vi "rsscope_core_global.vi"() -> ()   [LabVIEW 2014] (continued)
"Range Table"="rsscope_rngNqEq", "Read Callback"="", "Write Callback"="", "Supported Models"="", "Instrument Options"="", "Flags"=0, "Help"="Selects the operator for the MISO and MOSI pattern.\n\nAvailable Repeated Capabilities:\nTrigger: TrigA, TrigB, TrigR\r\n\nRemote-control command(s):\nTRIGger<m>:SPI:FCONdition"}, {"Level"=3, "Class Only"=FALSE, "Identifier"="RSSCOPE_ATTR_PROTOCOL_SPI_TRIGGER_MOSI_PATTERN", "Descriptive Name"="Protocol SPI Trigger MOSI Pattern", "Data Type"=2, "Command"="TRIG{Trigger}:SPI:MOS", "Access"=2, "Range Table"="", "Read Callback"="", "Write Callback"="", "Supported Models"="", "Instrument Options"="", "Flags"=0, "Help"="Specifies the pattern to be triggered on the MOSI line.\n\nAvailable Repeated Capabilities:\nTrigger: TrigA, TrigB, TrigR\r\n\nRemote-control command(s):\nTRIGger<m>:SPI:MOSipattern"}, {"Level"=3, "Class Only"=FALSE, "Identifier"="RSSCOPE_ATTR_PROTOCOL_SPI_TRIGGER_MISO_PATTERN", "Descriptive Name"="Protocol SPI Trigger MISO Pattern", "Data Type"=2, "Command"="TRIG{Trigger}:SPI:MIS", "Access"=2, "Range Table"="", "Read Callback"="", "Write Callback"="", "Supported Models"="", "Instrument Options"="", "Flags"=0, "Help"="Specifies the pattern to be triggered on the MOSI line.\n\nAvailable Repeated Capabilities:\nTrigger: TrigA, TrigB, TrigR\r\n\nRemote-control command(s):\nTRIGger<m>:SPI:MISopattern"}, {"Level"=2, "Class Only"=TRUE, "Identifier"="", "Descriptive Name"="UART", "Data Type"=0, "Command"="", "Access"=0, "Range Table"="", "Read Callback"="", "Write Callback"="", "Supported Models"="", "Instrument Options"="", "Flags"=0, "Help"="Configures UART trigger settings."}, {"Level"=3, "Class Only"=FALSE, "Identifier"="RSSCOPE_ATTR_PROTOCOL_UART_TRIGGER_MODE", "Descriptive Name"="Protocol UART Trigger Mode", "Data Type"=0, "Command"="TRIG{Trigger}:UART:TYPE", "Access"=2, "Range Table"="rsscope_rngProtocolUARTTriggerType", "Read Callback"="", "Write Callback"="", "Supported Models"="", "Instrument Options"="", "Flags"=0, "Help"="Selects the trigger type for UART analysis.\n\nAvailable Repeated Capabilities:\nTrigger: TrigA, TrigB, TrigR\r\n\nRemote-control command(s):\nTRIGger<m>:UART:TYPE"}, {"Level"=3, "Class Only"=FALSE, "Identifier"="RSSCOPE_ATTR_PROTOCOL_UART_TRIGGER_SOURCE", "Descriptive Name"="Protocol UART Trigger Source", "Data Type"=0, "Command"="TRIG{Trigger}:UART:SOUR", "Access"=2, "Range Table"="rsscope_rngProtocolUARTLine", "Read Callback"="", "Write Callback"="", "Supported Models"="", "Instrument Options"="", "Flags"=0, "Help"="Selects the transmitter or receiver line as trigger source.\n\nAvailable Repeated Capabilities:\nTrigger: TrigA, TrigB, TrigR\r\n\nRemote-control command(s):\nTRIGger<m>:UART:SOURce"}, {"Level"=3, "Class Only"=FALSE, "Identifier"="RSSCOPE_ATTR_PROTOCOL_UART_TRIGGER_DATA_PATTERN", "Descriptive Name"="Protocol UART Trigger Data Pattern", "Data Type"=2, "Command"="TRIG{Trigger}:UART:DATA", "Access"=2, "Range Table"="", "Read Callback"="", "Write Callback"="", "Supported Models"="", "Instrument Options"="", "Flags"=0, "Help"="Specifies the data pattern to be found on the specified trigger source, in bin format. Enter the words in msb first bit order.\n\nAvailable Repeated Capabilities:\nTrigger: TrigA, TrigB, TrigR\r\n\nRemote-control command(s):\nTRIGger<m>:UART:DATA"}, {"Level"=3, "Class Only"=FALSE, "Identifier"="RSSCOPE_ATTR_PROTOCOL_UART_TRIGGER_DATA_PATTERN_CONDITION", "Descriptive Name"="Protocol UART Trigger Data Pattern Condition", "Data Type"=0, "Command"="TRIG{Trigger}:UART:FCON", "Access"=2, "Range Table"="rsscope_rngProtocolUARTDataOperator", "Read Callback"="", "Write Callback"="", "Supported Models"="", "Instrument Options"="", "Flags"=0, "Help"="Selects the operator for the data pattern.\n\nAvailable Repeated Capabilities:\nTrigger: TrigA, TrigB, TrigR\r\n\nRemote-control command(s):\nTRIGger<m>:UART:FCONdition"}, {"Level"=3, "Class Only"=FALSE, "Identifier"="RSSCOPE_ATTR_PROTOCOL_UART_TRIGGER_DATA_POSITION", "Descriptive Name"="Protocol UART Trigger Data Position", "Data Type"=0, "Command"="TRIG{Trigger}:UART:DPOP", "Access"=2, "Range Table"="rsscope_rngProtocolUARTDataPosition", "Read Callback"="", "Write Callback"="", "Supported Models"="", "Instrument Options"="", "Flags"=0, "Help"="Sets the operator for the data position. You can defined an exact position, or a position range.\n\nAvailable Repeated Capabilities:\nTrigger: TrigA, TrigB, TrigR\r\n\nRemote-control command(s):\nTRIGger<m>:UART:DPOPerator"}, {"Level"=3, "Class Only"=FALSE, "Identifier"="RSSCOPE_ATTR_PROTOCOL_UART_TRIGGER_DATA_POSITION_INDEX_MIN", "Descriptive Name"="Protocol UART Trigger Data Position Index Min", "Data Type"=0, "Command"="TRIG{Trigger}:UART:DPOS", "Access"=2, "Range Table"="rsscope_rngProtocolUARTDataIndexMin", "Read Callback"="", "Write Callback"="", "Supported Models"="", "Instrument Options"="", "Flags"=0, "Help"="Sets the number of words before the first word of interest. These offset words are ignored.\n\nAvailable Repeated Capabilities:\nTrigger: TrigA, TrigB, TrigR\r\n\nRemote-control command(s):\nTRIGger<m>:UART:DPOSition"}, {"Level"=3, "Class Only"=FALSE, "Identifier"="RSSCOPE_ATTR_PROTOCOL_UART_TRIGGER_DATA_POSITION_INDEX_MAX", "Descriptive Name"="Protocol UART Trigger Data Position Index Max", "Data Type"=0, "Command"="TRIG:UART:DPTO", "Access"=2, "Range Table"="rsscope_rngProtocolUARTDataIndexMax", "Read Callback"="", "Write Callback"="", "Supported Models"="", "Instrument Options"="", "Flags"=0, "Help"="Defines the last word of interest, if  RSSCOPE_ATTR_PROTOCOL_UART_TRIGGER_DATA_POSITION \ndefines a position range.\n\nAvailable Repeated Capabilities:\nNone\n\nRemote-control command(s):\nTRIGger<m>:UART:DPTO"}, {"Level"=2, "Class Only"=TRUE, "Identifier"="", "Descriptive Name"="LIN", "Data Type"=0, "Command"="", "Access"=0, "Range Table"="", "Read Callback"="", "Write Callback"="", "Supported Models"="", "Instrument Options"="", "Flags"=0, "Help"="Configures LIN trigger settings."}, {"Level"=3, "Class Only"=FALSE, "Identifier"="RSSCOPE_ATTR_PROTOCOL_LIN_TRIGGER_MODE", "Descriptive Name"="Protocol LIN Trigger Mode", "Data Type"=0, "Command"="TRIG{Trigger}:LIN:TYPE", "Access"=2, "Range Table"="rsscope_rngProtocolLINTrigger", "Read Callback"="", "Write Callback"="", "Supported Models"="", "Instrument Options"="K0|K3", "Flags"=0, "Help"="Selects the trigger type for LIN analysis.\n\nAvailable Repeated Capabilities:\nTrigger: TrigA, TrigB, TrigR\r\n\nRemote-control command(s):\nTRIGger<m>:LIN:TYPE"}, {"Level"=3, "Class Only"=FALSE, "Identifier"="RSSCOPE_ATTR_PROTOCOL_LIN_TRIGGER_DATA_CONDITION", "Descriptive Name"="Protocol LIN Trigger Data Condition", "Data Type"=0, "Command"="TRIG{Trigger}:LIN:DLEC", "Access"=2, "Range Table"="rsscope_rngProtocolLINTriggerDataCondition", "Read Callback"="", "Write Callback"="", "Supported Models"="", "Instrument Options"="", "Flags"=0, "Help"="Sets the operator to set the data length code for triggering on LIN data. For big endian transfer direction, you can trigger on a number of bytes less than the data length of the frame, that means, on the beginning of the data pattern. For little endian transfer direction, the exact number of data bytes in the frame must be set.\n\nAvailable Repeated Capabilities:\nTrigger: TrigA, TrigB, TrigR\r\n\nRemote-control command(s):\nTRIGger<m>:LIN:DLECondition"}, {"Level"=3, "Class Only"=FALSE, "Identifier"="RSSCOPE_ATTR_PROTOCOL_LIN_TRIGGER_DATA_LENGTH", "Descriptive Name"="Protocol LIN Trigger Data Length", "Data Type"=0, "Command"="TRIG{Trigger}:LIN:DLEN", "Access"=2, "Range Table"="rsscope_rngLINDataLength", "Read Callback"="", "Write Callback"="", "Supported Models"="", "Instrument Options"="", "Flags"=0, "Help"="Sets the length of the bit pattern to be found, in bytes. For &apos;Big Endian&apos; transfer direction, you can trigger on a number of bytes less than the data length of the frame, that means, on the beginning of the data pattern. For &apos;Little Endian&apos; transfer direction, the exact number of data bytes in the frame must be set.\n\nAvailable Repeated Capabilities:\nTrigger: TrigA, TrigB, TrigR\r\n\nRemote-control command(s):\nTRIGger<m>:LIN:DLENgth"}, {"Level"=3, "Class Only"=FALSE, "Identifier"="RSSCOPE_ATTR_PROTOCOL_LIN_TRIGGER_DATA_TRANSFER", "Descriptive Name"="Protocol LIN Trigger Data Transfer", "Data Type"=0, "Command"="TRIG{Trigger}:LIN:BORD", "Access"=2, "Range Table"="rsscope_rngLINDataTransfer", "Read Callback"="", "Write Callback"="", "Supported Models"="", "Instrument Options"="", "Flags"=0, "Help"="Sets the byte order (endianess) of the data transfer. According to the standard, LIN data is transmitted in little endian transfer order.\n\nAvailable Repeated Capabilities:\nTrigger: TrigA, TrigB, TrigR\r\n\nRemote-control command(s):\nTRIGger<m>:LIN:BORDer"}, {"Level"=3, "Class Only"=TRUE, "Identifier"="", "Descriptive Name"="Data", "Data Type"=0, "Command"="", "Access"=0, "Range Table"="", "Read Callback"="", "Write Callback"="", "Supported Models"="", "Instrument Options"="", "Flags"=0, "Help"="Configures data setup."}, {"Level"=4, "Class Only"=FALSE, "Identifier"="RSSCOPE_ATTR_PROTOCOL_LIN_TRIGGER_CONDITION_DATA", "Descriptive Name"="Protocol LIN Trigger Condition Data", "Data Type"=0, "Command"="TRIG{Trigger}:LIN:DCON", "Access"=2, "Range Table"="rsscope_rngProtocolTriggerCondition", "Read Callback"="", "Write Callback"="", "Supported Models"="", "Instrument Options"="", "Flags"=0, "Help"="Sets the operator to set a specific data or an data range.\n\nAvailable Repeated Capabilities:\nTrigger: TrigA, TrigB, TrigR\r\n\nRemote-control command(s):\nTRIGger<m>:LIN:DCONdition"}, {"Level"=4, "Class Only"=FALSE, "Identifier"="RSSCOPE_ATTR_PROTOCOL_LIN_TRIGGER_PATTERN_DATA_MIN", "Descriptive Name"="Protocol LIN Trigger Pattern Data Min", "Data Type"=2, "Command"="TRIG{Trigger}:LIN:DMIN", "Access"=2, "Range Table"="", "Read Callback"="", "Write Callback"="", "Supported Models"="", "Instrument Options"="", "Flags"=0, "Help"="Sets the trigger pattern, or sets the start value of an pattern range.\n\nNote(s):\n\n(1) Valid values 1; 0; or X (any bit), use of X is restricted to the conditions &apos;Equal&apos; and &apos;Not equal&apos;.\n\n(2) Data binary pattern string consist 8 Bytes.\n\nAvailable Repeated Capabilities:\nTrigger: TrigA, TrigB, TrigR\r\n\nRemote-control command(s):\nTRIGger<m>:LIN:DMIN"}, {"Level"=4, "Class Only"=FALSE, "Identifier"="RSSCOPE_ATTR_PROTOCOL_LIN_TRIGGER_PATTERN_DATA_MAX", "Descriptive Name"="Protocol LIN Trigger Pattern Data Max", "Data Type"=2, "Command"="TRIG{Trigger}:LIN:DMAX", "Access"=2, "Range Table"="", "Read Callback"="", "Write Callback"="", "Supported Models"="", "Instrument Options"="", "Flags"=0, "Help"="Sets the end value of trigger pattern range if condition is &apos;In range&apos; and &apos;Out of range&apos; (see RSSCOPE_ATTR_PROTOCOL_LIN_TRIGGER_CONDITION).\n \nNote(s):\n(1) Valid values 1; 0; or X (any bit), use of X is restricted to the conditions &apos;Equal&apos; and &apos;Not equal&apos;.\n\n(2) Data binary pattern string consist 8 Bytes.\n\nAvailable Repeated Capabilities:\nTrigger: TrigA, TrigB, TrigR\r\n\nRemote-control command(s):\nTRIGger<m>:LIN:DMAX"}, {"Level"=3, "Class Only"=TRUE, "Identifier"="", "Descriptive Name"="Identifier", "Data Type"=0, "Command"="", "Access"=0, "Range Table"="", "Read Callback"="", "Write Callback"="", "Supported Models"="", "Instrument Options"="", "Flags"=0, "Help"="Configures identifier setup."}, {"Level"=4, "Class Only"=FALSE, "Identifier"="RSSCOPE_ATTR_PROTOCOL_LIN_TRIGGER_IDENTIFIER_CONDITION", "Descriptive Name"="Protocol LIN Trigger Identifier Condition", "Data Type"=0, "Command"="TRIG{Trigger}:LIN:ICON", "Access"=2, "Range Table"="rsscope_rngProtocolTriggerCondition", "Read Callback"="", "Write Callback"="", "Supported Models"="", "Instrument Options"="", "Flags"=0, "Help"="Sets the operator to set a specific identifier or an identifier range.\n\nAvailable Repeated Capabilities:\nTrigger: TrigA, TrigB, TrigR\r\n\nRemote-control command(s):\nTRIGger<m>:LIN:ICONdition"}, {"Level"=4, "Class Only"=FALSE, "Identifier"="RSSCOPE_ATTR_PROTOCOL_LIN_TRIGGER_PATTERN_IDENTIFIER_MIN", "Descriptive Name"="Protocol LIN Trigger Pattern Identifier Min", "Data Type"=2, "Command"="TRIG{Trigger}:LIN:IMIN", "Access"=2, "Range Table"="", "Read Callback"="", "Write Callback"="", "Supported Models"="", "Instrument Options"="", "Flags"=0, "Help"="Sets the trigger pattern, or sets the start value of an pattern range.\n\nNote(s):\n\n(1) Valid values 1; 0; or X (any bit), use of X is restricted to the conditions &apos;Equal&apos; and &apos;Not equal&apos;.\n\n(2) ID binary pattern string consist 6 bits.\n\nAvailable Repeated Capabilities:\nTrigger: TrigA, TrigB, TrigR\r\n\nRemote-control command(s):\nTRIGger<m>:LIN:IMIN"}, {"Level"=4, "Class Only"=FALSE, "Identifier"="RSSCOPE_ATTR_PROTOCOL_LIN_TRIGGER_PATTERN_IDENTIFIER_MAX", "Descriptive Name"="Protocol LIN Trigger Pattern Identifier Max", "Data Type"=2, "Command"="TRIG{Trigger}:LIN:IMAX", "Access"=2, "Range Table"="", "Read Callback"="", "Write Callback"="", "Supported Models"="", "Instrument Options"="", "Flags"=0, "Help"="Sets the end value of trigger pattern range if condition is &apos;In range&apos; and &apos;Out of range&apos; (see RSSCOPE_ATTR_PROTOCOL_LIN_TRIGGER_CONDITION).\n \nNote(s):\n(1) Valid values 1; 0; or X (any bit), use of X is restricted to the conditions &apos;Equal&apos; and &apos;Not equal&apos;.\n\n(2) ID binary pattern string consist 6 bits.\n\nAvailable Repeated Capabilities:\nTrigger: TrigA, TrigB, TrigR\r\n\nRemote-control command(s):\nTRIGger<m>:LIN:IMAX"}, {"Level"=3, "Class Only"=TRUE, "Identifier"="", "Descriptive Name"="OR Slot", "Data Type"=0, "Command"="", "Access"=0, "Range Table"="", "Read Callback"="", "Write Callback"="", "Supported Models"="", "Instrument Options"="", "Flags"=0, "Help"="Sets the trigger to a combination of up to four identifiers. Enter the patterns in the &apos;Frame\nID&apos; fields. In binary and hex format, characters 1, 0, and X (don&apos;t care) are allowed. For\neach identifier pattern to be triggered on, enable &apos;Monitor&apos;."}, {"Level"=4, "Class Only"=FALSE, "Identifier"="RSSCOPE_ATTR_PROTOCOL_LIN_TRIGGER_ADDRESS_OR_STATE", "Descriptive Name"="Protocol LIN Trigger Address OR State", "Data Type"=3, "Command"="TRIG{Trigger}:LIN:IDOR{ORSlot}:ENAB", "Access"=2, "Range Table"="", "Read Callback"="", "Write Callback"="", "Supported Models"="", "Instrument Options"="K0|K3", "Flags"=2, "Help"="If set to &apos;On&apos; the indicated ADOR address is included in the &apos;identifier OR&apos; trigger condition.\n\nAvailable Repeated Capabilities:\nTrigger: TrigA, TrigB, TrigR\r\nORSlot: ORSlot1, ORSlot2, ORSlot3, ORSlot4\r\n\nRemote-control command(s):\nTRIGger<m>:LIN:IDOR<n>:ENABle"}, {"Level"=4, "Class Only"=FALSE, "Identifier"="RSSCOPE_ATTR_PROTOCOL_LIN_TRIGGER_ADDRESS_OR", "Descriptive Name"="Protocol LIN Trigger Address OR", "Data Type"=2, "Command"="TRIG{Trigger}:LIN:IDOR{ORSlot}", "Access"=2, "Range Table"="", "Read Callback"="", "Write Callback"="", "Supported Models"="", "Instrument Options"="K0|K3", "Flags"=0, "Help"="Sets the pattern of the indicated IDOR identifier in the &apos;identifier OR&apos; trigger condition.\n\nValid Values: \nBinary pattern string consisting bits of 1; 0; or X (any bit).\n\nAvailable Repeated Capabilities:\nTrigger: TrigA, TrigB, TrigR\r\nORSlot: ORSlot1, ORSlot2, ORSlot3, ORSlot4\r\n\nRemote-control command(s):\nTRIGger<m>:LIN:IDOR<n>[:VALue]"}, {"Level"=3, "Class Only"=TRUE, "Identifier"="", "Descriptive Name"="Error Conditions", "Data Type"=0, "Command"="", "Access"=0, "Range Table"="", "Read Callback"="", "Write Callback"="", "Supported Models"="", "Instrument Options"="", "Flags"=0, "Help"="Triggers if one or more of the following errors occur: Checksum error, Identifier parity error, Sync error."}, {"Level"=4, "Class Only"=FALSE, "Identifier"="RSSCOPE_ATTR_PROTOCOL_LIN_TRIGGER_CHECKSUM_ERROR", "Descriptive Name"="Protocol LIN Trigger Checksum Error", "Data Type"=3, "Command"="TRIG{Trigger}:LIN:CHKS", "Access"=2, "Range Table"="", "Read Callback"="", "Write Callback"="", "Supported Models"="", "Instrument Options"="", "Flags"=0, "Help"="This attribute configures conditions for Error Condition trigger. It&apos;s possible trigger on CRC Error.\n\nAvailable Repeated Capabilities:\nTrigger: TrigA, TrigB, TrigR\r\n\nRemote-control command(s):\nTRIGger<m>:LIN:CHKSerror"}, {"Level"=4, "Class Only"=FALSE, "Identifier"="RSSCOPE_ATTR_PROTOCOL_LIN_TRIGGER_CRC_ERROR_PATTERN", "Descriptive Name"="Protocol LIN Trigger CRC Error Pattern", "Data Type"=2, "Command"="TRIG{Trigger}:LIN:ERRP", "Access"=2, "Range Table"="", "Read Callback"="", "Write Callback"="", "Supported Models"="", "Instrument Options"="K0|K3", "Flags"=0, "Help"="Sets bit pattern of the slave identifier (&apos;ID&apos;).\n\nValid Values: \nBinary pattern string consisting 1; 0; or X (any bit).\n\nAvailable Repeated Capabilities:\nTrigger: TrigA, TrigB, TrigR\r\n\nRemote-control command(s):\nTRIGger<m>:LIN:ERRPattern"}, {"Level"=4, "Class Only"=FALSE, "Identifier"="RSSCOPE_ATTR_PROTOCOL_LIN_TRIGGER_CRC_ERROR_DATA_LENGTH", "Descriptive Name"="Protocol LIN Trigger CRC Error Data Length", "Data Type"=0, "Command"="TRIG{Trigger}:LIN:CRCD", "Access"=2, "Range Table"="rsscope_rngLINTriggerCRCErrDataLength", "Read Callback"="", "Write Callback"="", "Supported Models"="", "Instrument Options"="K0|K3", "Flags"=0, "Help"="Sets the number of data bytes to trigger on CRC errors.\n\nAvailable Repeated Capabilities:\nTrigger: TrigA, TrigB, TrigR\r\n\nRemote-control command(s):\nTRIGger<m>:LIN:CRCDatalen"}, {"Level"=4, "Class Only"=FALSE, "Identifier"="RSSCOPE_ATTR_PROTOCOL_LIN_TRIGGER_CRC_STANDARD", "Descriptive Name"="Protocol LIN Trigger CRC Standard", "Data Type"=0, "Command"="TRIG{Trigger}:LIN:STAN", "Access"=2, "Range Table"="rsscope_rngProtocolLINTriggerCRCStandard", "Read Callback"="", "Write Callback"="", "Supported Models"="", "Instrument Options"="", "Flags"=0, "Help"="Sets the LIN standard to trigger on CRC errors.\n\nAvailable Repeated Capabilities:\nTrigger: TrigA, TrigB, TrigR\r\n\nRemote-control command(s):\nTRIGger<m>:LIN:STANdard"}, {"Level"=4, "Class Only"=FALSE, "Identifier"="RSSCOPE_ATTR_PROTOCOL_LIN_TRIGGER_IDENTIFIER_PARITY_ERROR", "Descriptive Name"="Protocol LIN Trigger Identifier Parity Error", "Data Type"=3, "Command"="TRIG{Trigger}:LIN:IPER", "Access"=2, "Range Table"="", "Read Callback"="", "Write Callback"="", "Supported Models"="", "Instrument Options"="", "Flags"=0, "Help"="Triggers if an error occurs in the identifier parity bits. These are the bits 6 and 7 of the\nidentifier.\n\nAvailable Repeated Capabilities:\nTrigger: TrigA, TrigB, TrigR\r\n\nRemote-control command(s):\nTRIGger<m>:LIN:IPERror"}, {"Level"=4, "Class Only"=FALSE, "Identifier"="RSSCOPE_ATTR_PROTOCOL_LIN_TRIGGER_SYNC_ERROR", "Descriptive Name"="Protocol LIN Trigger Sync Error", "Data Type"=3, "Command"="TRIG{Trigger}:LIN:SYER", "Access"=2, "Range Table"="", "Read Callback"="", "Write Callback"="", "Supported Models"="", "Instrument Options"="", "Flags"=0, "Help"="Triggers if a synchronization error occurs.\n\nAvailable Repeated Capabilities:\nTrigger: TrigA, TrigB, TrigR\r\n\nRemote-control command(s):\nTRIGger<m>:LIN:SYERror"}, {"Level"=2, "Class Only"=TRUE, "Identifier"="", "Descriptive Name"="CAN", "Data Type"=0, "Command"="", "Access"=0, "Range Table"="", "Read Callback"="", "Write Callback"="", "Supported Models"="", "Instrument Options"="", "Flags"=0, "Help"="Configures CAN trigger settings."}, {"Level"=3, "Class Only"=FALSE, "Identifier"="RSSCOPE_ATTR_PROTOCOL_CAN_TRIGGER_MODE", "Descriptive Name"="Protocol CAN Trigger Mode", "Data Type"=0, "Command"="TRIG{Trigger}:CAN:TYPE", "Access"=2, "Range Table"="rsscope_rngProtocolCANTriggMode", "Read Callback"="", "Write Callback"="", "Supported Models"="", "Instrument Options"="K0|K3", "Flags"=0, "Help"="Selects the trigger type for CAN analysis.\n\nAvailable Repeated Capabilities:\nTrigger: TrigA, TrigB, TrigR\r\n\nRemote-control command(s):\nTRIGger<m>:CAN:TYPE"}, {"Level"=3, "Class Only"=FALSE, "Identifier"="RSSCOPE_ATTR_PROTOCOL_CAN_TRIGGER_FRAME_TYPE", "Descriptive Name"="Protocol CAN Trigger Frame Type", "Data Type"=0, "Command"="TRIG{Trigger}:CAN:FTYP", "Access"=2, "Range Table"="rsscope_rngProtocolCANTriggFrameType", "Read Callback"="", "Write Callback"="", "Supported Models"="", "Instrument Options"="K0|K3", "Flags"=0, "Help"="Selects the frame type which will be used as trigger condition when trigger mode is set to &apos;Frame Type&apos; (see RSSCOPE_ATTR_PROTOCOL_CAN_TRIGGER_MODE)\n\nAvailable Repeated Capabilities:\nTrigger: TrigA, TrigB, TrigR\r\n\nRemote-control command(s):\nTRIGger<m>:CAN:FTYPe"}, {"Level"=3, "Class Only"=FALSE, "Identifier"="RSSCOPE_ATTR_PROTOCOL_CAN_TRIGGER_STANDARD", "Descriptive Name"="Protocol CAN Trigger Standard", "Data Type"=0, "Command"="TRIG{Trigger}:CAN:FDAT:STAN", "Access"=2, "Range Table"="rsscope_rngCANStandard", "Read Callback"="", "Write Callback"="", "Supported Models"="", "Instrument Options"="K9", "Flags"=0, "Help"="Selects the CAN standard. Use ANY if the standard of the signal is unknown.\n\nAvailable Repeated Capabilities:\nTrigger: TrigA, TrigB, TrigR\r\n\nRemote-control command(s):\nTRIGger<m>:CAN:FDATa:STANdard"}, {"Level"=3, "Class Only"=FALSE, "Identifier"="RSSCOPE_ATTR_PROTOCOL_CAN_TRIGGER_ID_TYPE", "Descriptive Name"="Protocol CAN Trigger ID Type", "Data Type"=0, "Command"="TRIG{Trigger}:CAN:ITYP", "Access"=2, "Range Table"="rsscope_rngProtocolCANIDType", "Read Callback"="", "Write Callback"="", "Supported Models"="", "Instrument Options"="K0|K3", "Flags"=0, "Help"="Selects the format of data and remote frames.\n\nAvailable Repeated Capabilities:\nTrigger: TrigA, TrigB, TrigR\r\n\nRemote-control command(s):\nTRIGger<m>:CAN:ITYPe"}, {"Level"=3, "Class Only"=FALSE, "Identifier"="RSSCOPE_ATTR_PROTOCOL_CAN_TRIGGER_FD_BITS_FDF", "Descriptive Name"="Protocol CAN Trigger FD Bits FDF", "Data Type"=0, "Command"="TRIG{Trigger}:CAN:FDAT:FDF", "Access"=2, "Range Table"="rsscope_rngCANFDBits", "Read Callback"="", "Write Callback"="", "Supported Models"="", "Instrument Options"="", "Flags"=0, "Help"="Specifies the CAN FD frame format. It corresponds to the EDL bit (extended data length), which only exists in CAN FD format.\n\nAvailable Repeated Capabilities:\nTrigger: TrigA, TrigB, TrigR\r\n\nRemote-control command(s):\nTRIGger<m>:CAN:FDATa:FDF"}, {"Level"=3, "Class Only"=FALSE, "Identifier"="RSSCOPE_ATTR_PROTOCOL_CAN_TRIGGER_FD_BITS_BRS", "Descriptive Name"="Protocol CAN Trigger FD Bits BRS", "Data Type"=0, "Command"="TRIG{Trigger}:CAN:FDAT:BRS", "Access"=2, "Range Table"="rsscope_rngCANFDBitRS", "Read Callback"="", "Write Callback"="", "Supported Models"="", "Instrument Options"="", "Flags"=0, "Help"="Sets the bit rate switch bit.\n\nAvailable Repeated Capabilities:\nTrigger: TrigA, TrigB, TrigR\r\n\nRemote-control command(s):\nTRIGger<m>:CAN:FDATa:BRS"}, {"Level"=3, "Class Only"=FALSE, "Identifier"="RSSCOPE_ATTR_PROTOCOL_CAN_TRIGGER_FD_BITS_ESI", "Descriptive Name"="Protocol CAN Trigger FD Bits ESI", "Data Type"=0, "Command"="TRIG{Trigger}:CAN:FDAT:ESI", "Access"=2, "Range Table"="rsscope_rngCANFDBits", "Read Callback"="", "Write Callback"="", "Supported Models"="", "Instrument Options"="", "Flags"=0, "Help"="Sets the error state indicator bit.\n\nAvailable Repeated Capabilities:\nTrigger: TrigA, TrigB, TrigR\r\n\nRemote-control command(s):\nTRIGger<m>:CAN:FDATa:ESI"}, {"Level"=3, "Class Only"=FALSE, "Identifier"="RSSCOPE_ATTR_PROTOCOL_CAN_TRIGGER_FRAME_ENDIANNESS", "Descriptive Name"="Protocol CAN Trigger Frame Endianness", "Data Type"=0, "Command"="TRIG{Trigger}:CAN:BORD", "Access"=2, "Range Table"="rsscope_rngProtocolCANEndianness", "Read Callback"="", "Write Callback"="", "Supported Models"="", "Instrument Options"="K0|K3", "Flags"=0, "Help"="Selects the byte order (endianness) of the data transfer.\n\nAvailable Repeated Capabilities:\nTrigger: TrigA, TrigB, TrigR\r\n\nRemote-control command(s):\nTRIGger<m>:CAN:BORDer"}, {"Level"=3, "Class Only"=TRUE, "Identifier"="", "Descriptive Name"="Data", "Data Type"=0, "Command"="", "Access"=0, "Range Table"="", "Read Callback"="", "Write Callback"="", "Supported Models"="", "Instrument Options"="", "Flags"=0, "Help"="Configures Trigger CAN data."}, {"Level"=4, "Class Only"=FALSE, "Identifier"="RSSCOPE_ATTR_PROTOCOL_CAN_TRIGGER_DATA_CONDITION", "Descriptive Name"="Protocol CAN Trigger Data Condition", "Data Type"=0, "Command"="TRIG{Trigger}:CAN:DCON", "Access"=2, "Range Table"="rsscope_rngProtocolTriggerCondition", "Read Callback"="", "Write Callback"="", "Supported Models"="", "Instrument Options"="", "Flags"=0, "Help"="Sets the operator to set a specific data pattern or a data pattern range.\n\nAvailable Repeated Capabilities:\nTrigger: TrigA, TrigB, TrigR\r\n\nRemote-control command(s):\nTRIGger<m>:CAN:DCONdition"}, {"Level"=4, "Class Only"=FALSE, "Identifier"="RSSCOPE_ATTR_PROTOCOL_CAN_TRIGGER_PATTERN_DATA_MIN", "Descriptive Name"="Protocol CAN Trigger Pattern Data Min", "Data Type"=2, "Command"="TRIG{Trigger}:CAN:DMIN", "Access"=2, "Range Table"="", "Read Callback"="", "Write Callback"="", "Supported Models"="", "Instrument Options"="", "Flags"=0, "Help"="Specifies a data pattern, or sets the start value of a data pattern range.\n\nAvailable Repeated Capabilities:\nTrigger: TrigA, TrigB, TrigR\r\n\nRemote-control command(s):\nTRIGger<m>:CAN:DMIN"}, {"Level"=4, "Class Only"=FALSE, "Identifier"="RSSCOPE_ATTR_PROTOCOL_CAN_TRIGGER_PATTERN_DATA_MAX", "Descriptive Name"="Protocol CAN Trigger Pattern Data Max", "Data Type"=2, "Command"="TRIG{Trigger}:CAN:DMAX", "Access"=2, "Range Table"="", "Read Callback"="", "Write Callback"="", "Supported Models"="", "Instrument Options"="", "Flags"=0, "Help"="Sets the end value of an data range.\n\nAvailable Repeated Capabilities:\nTrigger: TrigA, TrigB, TrigR\r\n\nRemote-control command(s):\nTRIGger<m>:CAN:DMAX"}, {"Level"=4, "Class Only"=FALSE, "Identifier"="RSSCOPE_ATTR_PROTOCOL_CAN_TRIGGER_DLC_CONDITION", "Descriptive Name"="Protocol CAN Trigger DLC Condition", "Data Type"=0, "Command"="TRIG{Trigger}:CAN:DLCC", "Access"=2, "Range Table"="RsScope_rngProtocolCANTriggerDLCCondition", "Read Callback"="", "Write Callback"="", "Supported Models"="", "Instrument Options"="", "Flags"=0, "Help"="Operator to set the data length code for triggering on CAN data. For big endian transfer direction, you can trigger on a number of bytes less than the DLC of the frame, that means, on the beginning of the data pattern. For little endian transfer direction, the exact number of data bytes in the frame must be set.\n\nAvailable Repeated Capabilities:\nTrigger: TrigA, TrigB, TrigR\r\n\nRemote-control command(s):\nTRIGger<m>:CAN:DLCCondition"}, {"Level"=4, "Class Only"=FALSE, "Identifier"="RSSCOPE_ATTR_PROTOCOL_CAN_TRIGGER_DLC", "Descriptive Name"="Protocol CAN Trigger DLC", "Data Type"=0, "Command"="TRIG{Trigger}:CAN:DLC", "Access"=2, "Range Table"="RsScope_rngProtocolCANTriggerDLC", "Read Callback"="", "Write Callback"="", "Supported Models"="", "Instrument Options"="", "Flags"=0, "Help"="Sets the Data Length Code, the number of data bytes to be found.\n\nAvailable Repeated Capabilities:\nTrigger: TrigA, TrigB, TrigR\r\n\nRemote-control command(s):\nTRIGger<m>:CAN:DLC"}, {"Level"=4, "Class Only"=FALSE, "Identifier"="RSSCOPE_ATTR_PROTOCOL_CAN_TRIGGER_NUMBER_OF_DATA_BYTES", "Descriptive Name"="Protocol CAN Trigger Number Of Data Bytes", "Data Type"=0, "Command"="TRIG{Trigger}:CAN:NDBY?", "Access"=0, "Range Table"="", "Read Callback"="", "Write Callback"="", "Supported Models"="", "Instrument Options"="K3", "Flags"=0, "Help"="Returns the number of data bytes defined by DLC. DLC and NDB are different in CAN FD for DLCs > 8.\n\nAvailable Repeated Capabilities:\nTrigger: TrigA, TrigB, TrigR\r\n\nRemote-control command(s):\nTRIGger<m>:CAN:NDBYtes?"}, {"Level"=4, "Class Only"=FALSE, "Identifier"="RSSCOPE_ATTR_PROTOCOL_CAN_TRIGGER_POSITION_CONDITION", "Descriptive Name"="Protocol CAN Trigger Position Condition", "Data Type"=0, "Command"="TRIG{Trigger}:CAN:FDAT:DPOP", "Access"=2, "Range Table"="rsscope_rngProtocolCANPositionCondition", "Read Callback"="", "Write Callback"="", "Supported Models"="", "Instrument Options"="K9", "Flags"=0, "Help"="Sets the operator to define an exact position or a data range where the instrument looks for the specified data pattern.\n\nAvailable Repeated Capabilities:\nTrigger: TrigA, TrigB, TrigR\r\n\nRemote-control command(s):\nTRIGger<m>:CAN:FDATa:DPOPerator"}, {"Level"=4, "Class Only"=FALSE, "Identifier"="RSSCOPE_ATTR_PROTOCOL_CAN_TRIGGER_POSITION_MIN", "Descriptive Name"="Protocol CAN Trigger Position Min", "Data Type"=0, "Command"="TRIG{Trigger}:CAN:FDAT:DPOS", "Access"=2, "Range Table"="rsscope_rngCANPositionMin", "Read Callback"="", "Write Callback"="", "Supported Models"="", "Instrument Options"="K9", "Flags"=0, "Help"="Defines the number of the first data byte at which the data pattern may start.\n\nAvailable Repeated Capabilities:\nTrigger: TrigA, TrigB, TrigR\r\n\nRemote-control command(s):\nTRIGger<m>:CAN:FDATa:DPOSition"}, {"Level"=4, "Class Only"=FALSE, "Identifier"="RSSCOPE_ATTR_PROTOCOL_CAN_TRIGGER_POSITION_MAX", "Descriptive Name"="Protocol CAN Trigger Position Max", "Data Type"=0, "Command"="TRIG{Trigger}:CAN:FDAT:DPTO", "Access"=2, "Range Table"="rsscope_rngCANPositionMax", "Read Callback"="", "Write Callback"="", "Supported Models"="", "Instrument Options"="K9", "Flags"=0, "Help"="Sets the number of the last byte at which the required data pattern may start.\n\nAvailable Repeated Capabilities:\nTrigger: TrigA, TrigB, TrigR\r\n\nRemote-control command(s):\nTRIGger<m>:CAN:FDATa:DPTO"}, {"Level"=3, "Class Only"=TRUE, "Identifier"="", "Descriptive Name"="Identifier", "Data Type"=0, "Command"="", "Access"=0, "Range Table"="", "Read Callback"="", "Write Callback"="", "Supported Models"="", "Instrument Options"="", "Flags"=0, "Help"="Configures trigger CAN identifier."}, {"Level"=4, "Class Only"=FALSE, "Identifier"="RSSCOPE_ATTR_PROTOCOL_CAN_TRIGGER_IDENTIFIER_CONDITION", "Descriptive Name"="Protocol CAN Trigger Identifier Condition", "Data Type"=0, "Command"="TRIG{Trigger}:CAN:ICON", "Access"=2, "Range Table"="rsscope_rngProtocolTriggerCondition", "Read Callback"="", "Write Callback"="", "Supported Models"="", "Instrument Options"="", "Flags"=0, "Help"="Sets the operator to set a specific identifier or an identifier range.\n\nAvailable Repeated Capabilities:\nTrigger: TrigA, TrigB, TrigR\r\n\nRemote-control command(s):\nTRIGger<m>:CAN:ICONdition"}, {"Level"=4, "Class Only"=FALSE, "Identifier"="RSSCOPE_ATTR_PROTOCOL_CAN_TRIGGER_PATTERN_IDENTIFIER_MIN", "Descriptive Name"="Protocol CAN Trigger Pattern Identifier Min", "Data Type"=2, "Command"="TRIG{Trigger}:CAN:IMIN", "Access"=2, "Range Table"="", "Read Callback"="", "Write Callback"="", "Supported Models"="", "Instrument Options"="", "Flags"=0, "Help"="Specifies a message identifier pattern, or sets the start value of an identifier range.\n\nAvailable Repeated Capabilities:\nTrigger: TrigA, TrigB, TrigR\r\n\nRemote-control command(s):\nTRIGger<m>:CAN:IMIN"}, {"Level"=4, "Class Only"=FALSE, "Identifier"="RSSCOPE_ATTR_PROTOCOL_CAN_TRIGGER_PATTERN_IDENTIFIER_MAX", "Descriptive Name"="Protocol CAN Trigger Pattern Identifier Max", "Data Type"=2, "Command"="TRIG{Trigger}:CAN:IMAX", "Access"=2, "Range Table"="", "Read Callback"="", "Write Callback"="", "Supported Models"="", "Instrument Options"="", "Flags"=0, "Help"="Sets the end value of an identifier range.\n\nAvailable Repeated Capabilities:\nTrigger: TrigA, TrigB, TrigR\r\n\nRemote-control command(s):\nTRIGger<m>:CAN:IMAX"}, {"Level"=3, "Class Only"=TRUE, "Identifier"="", "Descriptive Name"="Error Conditions", "Data Type"=0, "Command"="", "Access"=0, "Range Table"="", "Read Callback"="", "Write Callback"="", "Supported Models"="", "Instrument Options"="", "Flags"=0, "Help"="If a CAN detects a bit stuffing error, form error, or ack error, it transmits an error flag at the next bit. The R&S RTO detects errors in the message and triggers on these errors even if no CAN node sends an error flag."}, {"Level"=4, "Class Only"=FALSE, "Identifier"="RSSCOPE_ATTR_PROTOCOL_CAN_TRIGGER_CHECKSUM_ERROR", "Descriptive Name"="Protocol CAN Trigger Checksum Error", "Data Type"=3, "Command"="TRIG{Trigger}:CAN:CRC", "Access"=2, "Range Table"="", "Read Callback"="", "Write Callback"="", "Supported Models"="", "Instrument Options"="", "Flags"=0, "Help"="Triggers on CRC errors. A CRC error occurs when the CRC calculated by the receiver differs from the received value in the CRC sequence.\n\nAvailable Repeated Capabilities:\nTrigger: TrigA, TrigB, TrigR\r\n\nRemote-control command(s):\nTRIGger<m>:CAN:CRCerror"}, {"Level"=4, "Class Only"=FALSE, "Identifier"="RSSCOPE_ATTR_PROTOCOL_CAN_TRIGGER_BIT_STUFFING_ERROR", "Descriptive Name"="Protocol CAN Trigger Bit Stuffing Error", "Data Type"=3, "Command"="TRIG{Trigger}:CAN:BITS", "Access"=2, "Range Table"="", "Read Callback"="", "Write Callback"="", "Supported Models"="", "Instrument Options"="", "Flags"=0, "Help"="Triggers if astuff error occurs - when the 6th consecutive equal bit level in the mentioned fields is detected.\n\nAvailable Repeated Capabilities:\nTrigger: TrigA, TrigB, TrigR\r\n\nRemote-control command(s):\nTRIGger<m>:CAN:BITSterror"}, {"Level"=4, "Class Only"=FALSE, "Identifier"="RSSCOPE_ATTR_PROTOCOL_CAN_TRIGGER_FORM_ERROR", "Descriptive Name"="Protocol CAN Trigger Form Error", "Data Type"=3, "Command"="TRIG{Trigger}:CAN:FORM", "Access"=2, "Range Table"="", "Read Callback"="", "Write Callback"="", "Supported Models"="", "Instrument Options"="", "Flags"=0, "Help"="Triggers when a fixed-form bit field contains one or more illegal bits.\n\nAvailable Repeated Capabilities:\nTrigger: TrigA, TrigB, TrigR\r\n\nRemote-control command(s):\nTRIGger<m>:CAN:FORMerror"}, {"Level"=4, "Class Only"=FALSE, "Identifier"="RSSCOPE_ATTR_PROTOCOL_CAN_TRIGGER_ACK_ERROR", "Descriptive Name"="Protocol CAN Trigger Ack Error", "Data Type"=3, "Command"="TRIG{Trigger}:CAN:ACK", "Access"=2, "Range Table"="", "Read Callback"="", "Write Callback"="", "Supported Models"="", "Instrument Options"="", "Flags"=0, "Help"="Triggers when the transmitter does not receive an acknowledgment - a dominant bit during the Ack Slot.\n\nAvailable Repeated Capabilities:\nTrigger: TrigA, TrigB, TrigR\r\n\nRemote-control command(s):\nTRIGger<m>:CAN:ACKerror"}, {"Level"=4, "Class Only"=FALSE, "Identifier"="RSSCOPE_ATTR_PROTOCOL_CAN_TRIGGER_STUFF_COUNT_ERROR", "Descriptive Name"="Protocol CAN Trigger Stuff Count Error", "Data Type"=3, "Command"="TRIG{Trigger}:CAN:FDAT:SCER", "Access"=2, "Range Table"="", "Read Callback"="", "Write Callback"="", "Supported Models"="", "Instrument Options"="K3", "Flags"=0, "Help"="Triggers on stuff count errors. A stuff count error occurs if th received stuff count value does not match the value calculated from the own stuff bit count.\n\nAvailable Repeated Capabilities:\nTrigger: TrigA, TrigB, TrigR\r\n\nRemote-control command(s):\nTRIGger<m>:CAN:FDATa:SCERror"}, {"Level"=3, "Class Only"=TRUE, "Identifier"="", "Descriptive Name"="Symbolic", "Data Type"=0, "Command"="", "Access"=0, "Range Table"="", "Read Callback"="", "Write Callback"="", "Supported Models"="", "Instrument Options"="", "Flags"=0, "Help"="This class configures symbolic trigger."}, {"Level"=4, "Class Only"=FALSE, "Identifier"="RSSCOPE_ATTR_PROTOCOL_CAN_SYMBOLIC_TRIGGER_MESSAGE", "Descriptive Name"="Protocol CAN Symbolic Trigger Message", "Data Type"=2, "Command"="TRIG{Trigger}:CAN:SYMB:MSGV", "Access"=2, "Range Table"="", "Read Callback"="", "Write Callback"="", "Supported Models"="", "Instrument Options"="", "Flags"=0, "Help"="Sets the message to be triggered or searched for.\n\nAvailable Repeated Capabilities:\nTrigger: TrigA, TrigB, TrigR\r\n\nRemote-control command(s):\nTRIGger<m>:CAN:SYMBolic:MSGValue"}, {"Level"=4, "Class Only"=FALSE, "Identifier"="RSSCOPE_ATTR_PROTOCOL_CAN_SYMBOLIC_TRIGGER_ON_SIGNAL", "Descriptive Name"="Protocol CAN Symbolic Trigger On Signal", "Data Type"=3, "Command"="TRIG{Trigger}:CAN:SYMB:TSIG", "Access"=2, "Range Table"="", "Read Callback"="", "Write Callback"="", "Supported Models"="", "Instrument Options"="", "Flags"=0, "Help"="Enables the trigger on a specific signal value that is part of the selected message.\n\nAvailable Repeated Capabilities:\nTrigger: TrigA, TrigB, TrigR\r\n\nRemote-control command(s):\nTRIGger<m>:CAN:SYMBolic:TSIGnals"}, {"Level"=4, "Class Only"=FALSE, "Identifier"="RSSCOPE_ATTR_PROTOCOL_CAN_SYMBOLIC_TRIGGER_SIGNAL_VALUE", "Descriptive Name"="Protocol CAN Symbolic Trigger Signal Value", "Data Type"=2, "Command"="TRIG{Trigger}:CAN:SYMB:SIGV", "Access"=2, "Range Table"="", "Read Callback"="", "Write Callback"="", "Supported Models"="", "Instrument Options"="", "Flags"=0, "Help"="Sets the signal name to be triggered or searched for.\n\nAvailable Repeated Capabilities:\nTrigger: TrigA, TrigB, TrigR\r\n\nRemote-control command(s):\nTRIGger<m>:CAN:SYMBolic:SIGValue"}, {"Level"=4, "Class Only"=FALSE, "Identifier"="RSSCOPE_ATTR_PROTOCOL_CAN_SYMBOLIC_TRIGGER_SIGNAL_MIN", "Descriptive Name"="Protocol CAN Symbolic Trigger Signal Min", "Data Type"=1, "Command"="TRIG{Trigger}:CAN:SYMB:DMIN", "Access"=2, "Range Table"="", "Read Callback"="", "Write Callback"="", "Supported Models"="", "Instrument Options"="", "Flags"=0, "Help"="Defines the minimum data value of the signal.\n\nAvailable Repeated Capabilities:\nTrigger: TrigA, TrigB, TrigR\r\n\nRemote-control command(s):\nTRIGger<m>:CAN:SYMBolic:DMIN"}, {"Level"=4, "Class Only"=FALSE, "Identifier"="RSSCOPE_ATTR_PROTOCOL_CAN_SYMBOLIC_TRIGGER_SIGNAL_MAX", "Descriptive Name"="Protocol CAN Symbolic Trigger Signal Max", "Data Type"=1, "Command"="TRIG{Trigger}:CAN:SYMB:DMAX", "Access"=2, "Range Table"="", "Read Callback"="", "Write Callback"="", "Supported Models"="", "Instrument Options"="", "Flags"=0, "Help"="Defines the maximum data value of the signal. This value is required to specify a range if condition is &apos;In range&apos; or &apos;Out of range&apos;.\n\nAvailable Repeated Capabilities:\nTrigger: TrigA, TrigB, TrigR\r\n\nRemote-control command(s):\nTRIGger<m>:CAN:SYMBolic:DMAX"}, {"Level"=4, "Class Only"=FALSE, "Identifier"="RSSCOPE_ATTR_PROTOCOL_CAN_SYMBOLIC_TRIGGER_SIGNAL_ENUM_VALUE", "Descriptive Name"="Protocol CAN Symbolic Trigger Signal Enum Value", "Data Type"=0, "Command"="TRIG{Trigger}:CAN:SYMB:SGEV", "Access"=2, "Range Table"="", "Read Callback"="", "Write Callback"="", "Supported Models"="", "Instrument Options"="", "Flags"=0, "Help"="Sets a symbolic data value for signals with enumerated values.\n\nAvailable Repeated Capabilities:\nTrigger: TrigA, TrigB, TrigR\r\n\nRemote-control command(s):\nTRIGger<m>:CAN:SYMBolic:SGEValue"}, {"Level"=2, "Class Only"=TRUE, "Identifier"="", "Descriptive Name"="Flex Ray", "Data Type"=0, "Command"="", "Access"=0, "Range Table"="", "Read Callback"="", "Write Callback"="", "Supported Models"="", "Instrument Options"="", "Flags"=0, "Help"="Configures Flex Ray trigger settings."}, {"Level"=3, "Class Only"=FALSE, "Identifier"="RSSCOPE_ATTR_PROTOCOL_FLEXRAY_TRIGGER_TYPE", "Descriptive Name"="Protocol FlexRay Trigger Type", "Data Type"=0, "Command"="TRIG{Trigger}:FLXR:TYPE", "Access"=2, "Range Table"="rsscope_rngFlexRayTriggerType", "Read Callback"="", "Write Callback"="", "Supported Models"="", "Instrument Options"="K4", "Flags"=0, "Help"="Configures the trigger type for FlexRay analysis.\n\nAvailable Repeated Capabilities:\nTrigger: TrigA, TrigB, TrigR\r\n\nRemote-control command(s):\nTRIGger<m>:FLXRay:TYPE"}, {"Level"=3, "Class Only"=FALSE, "Identifier"="RSSCOPE_ATTR_PROTOCOL_FLEXRAY_TRIGGER_CYCLE_STEP", "Descriptive Name"="Protocol FlexRay Trigger Cycle Step", "Data Type"=0, "Command"="TRIG{Trigger}:FLXR:CST", "Access"=2, "Range Table"="rsscope_rngFlexRayCycleStep", "Read Callback"="", 
